vi "Timestamp to SQL Time.vi"(1 "seconds since 1Jan1904":timestamp) -> (0 "date/time string":string)   [LabVIEW 2013, in "Data.PGSQL.lvclass"]
uses:
  Data.PGSQL.lvclass
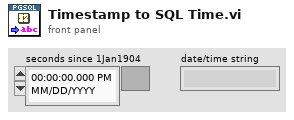
[diagram p1: front panel]
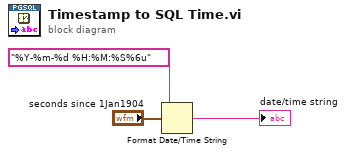
[diagram p0: block diagram]
diagram:
  n1 = Format Date/Time String(time format string (%c)="%Y-%m-%d %H:%M:%S%6u", seconds (now)="seconds since 1Jan1904") -> (date/time string=→"date/time string":string)  [unwired: 1 in]
